vi "QD_Main.vi"(0 "State_and_Data_In":T1, 1 "Max_Queue_Size_In":i32=-1, 2 "Queue_Name_In":string, 5 "State_and_Data_N_In":T1[](array[typedef]), 7 "Time_Out_In_ms (-1)":i32, 11 "Error_In":errorcluster, 13 "Queue_Operation":T2=enum."Flush") -> (4 "State_and_Data_Out":T1, 6 "State_and_Data_N_Out":T1[](array[typedef]), 15 "Error_Out":errorcluster)   [LabVIEW 2021]
doc: "Used to transfer data from one loop to another using queue."
uses:
  Controls/State_and_Data.ctl
  Controls/Queue_Operation.ctl
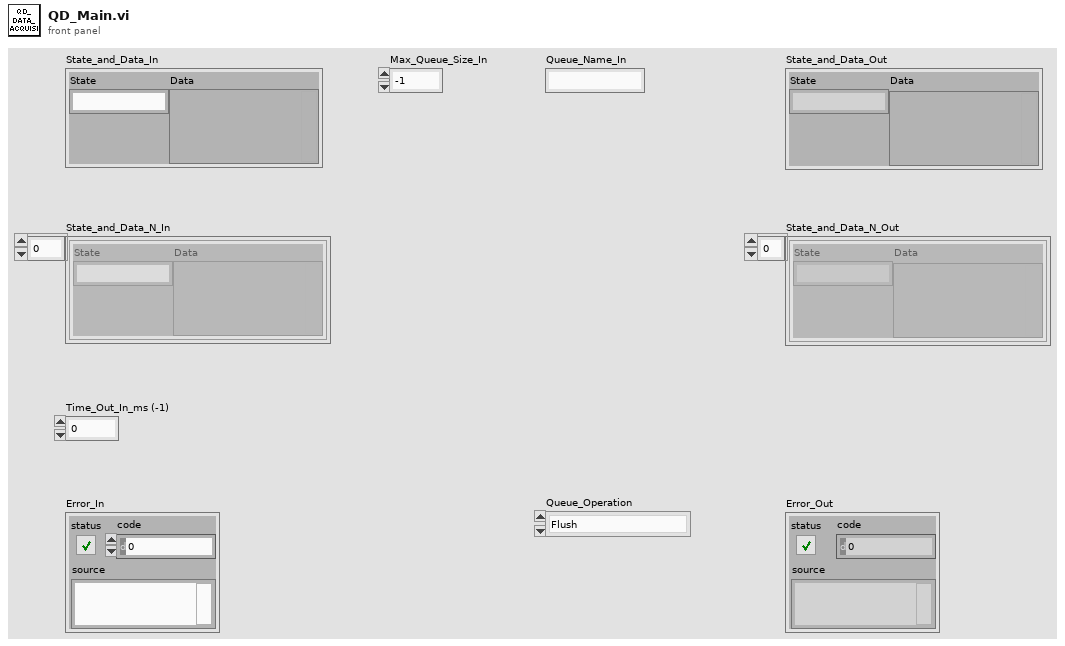
[diagram p1: front panel]
types:
  T1 = typedef "State_and_Data.ctl" = cluster{"State":string, "Data":variant}
  T2 = typedef "Queue_Operation.ctl" = enum16{"Obtain_Queue", "Enqueue", "Enqueue_First", "Enqueue_N", "Lossy_Enqueue", "Preview", "Queue_Status", "Dequeue", "Flush", "Release_Queue"}
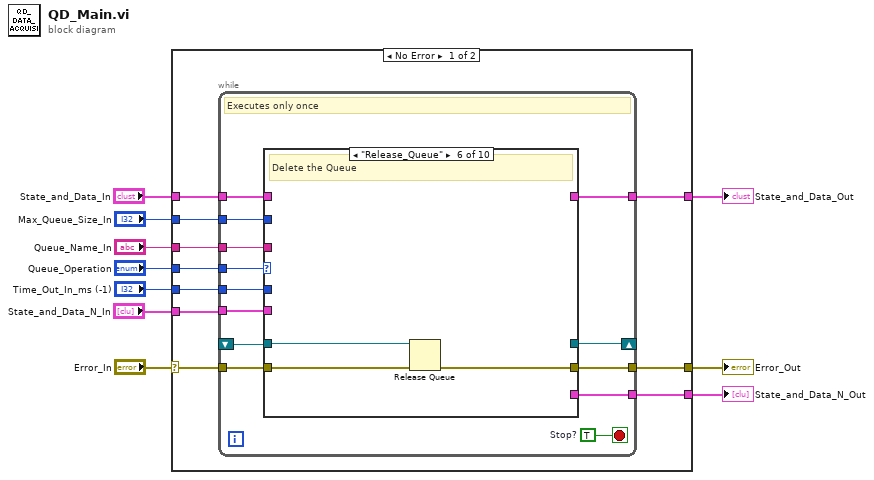
[diagram p0: block diagram]
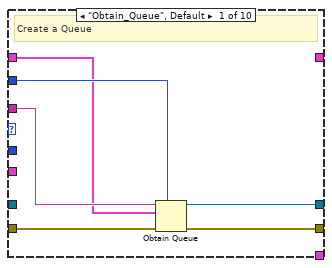
[diagram p2: hidden frame]
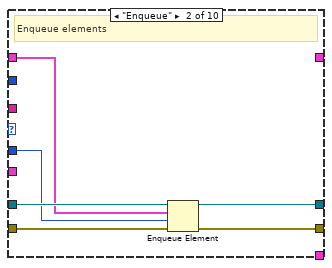
[diagram p3: hidden frame]
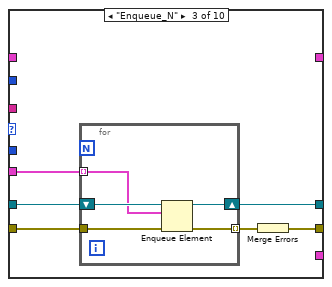
[diagram p4: hidden frame]
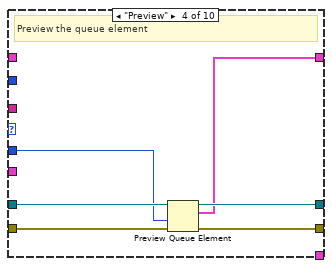
[diagram p5: hidden frame]
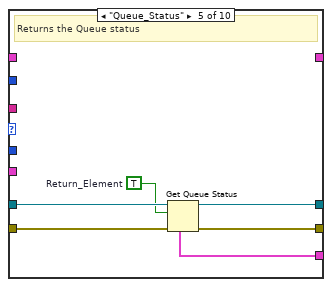
[diagram p6: hidden frame]
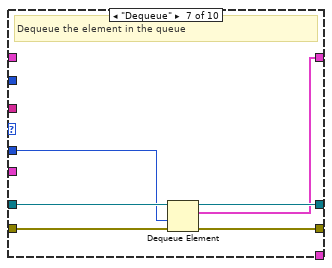
[diagram p7: hidden frame]
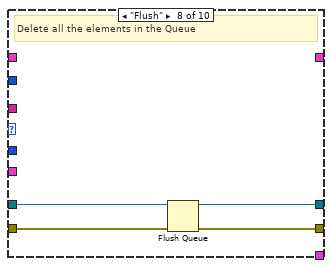
[diagram p8: hidden frame]
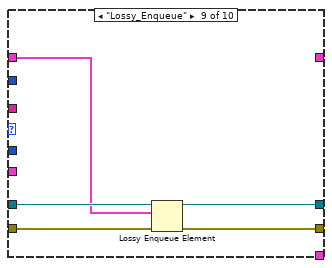
[diagram p9: hidden frame]
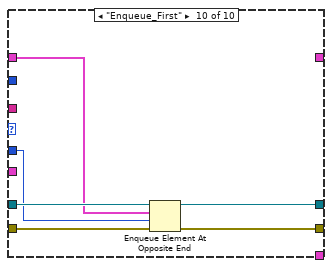
[diagram p10: hidden frame]
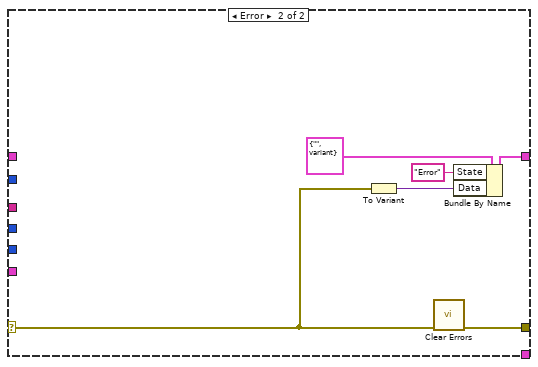
[diagram p11: hidden frame]
diagram:
  n1 = case shown="No Error" "Error_In" {
    selector: "Error_In" -> [w11 w95]
    tunnel: "Max_Queue_Size_In" -> [w20 _]
    tunnel: [w19 w98] -> w9
    tunnel: "Time_Out_In_ms (-1)" -> [w18 _]
    tunnel: "Queue_Operation" -> [w17 _]
    tunnel: "Queue_Name_In" -> [w16 _]
    tunnel: "State_and_Data_In" -> [w15 _]
    tunnel: [w14 w96] -> w4
    tunnel: [w13 _] -> w3
    tunnel: "State_and_Data_N_In" -> [w12 _]
    frame No Error {
      n2 = while {
        tunnel: w20 -> [w33]
        tunnel: w18 -> [w30]
        tunnel: w17 -> [w27]
        tunnel: [w25] -> w13
        shift-right: [w28] -> _
        shift-left: _ -> [w23]
        tunnel: w11 -> [w24]
        tunnel: [w32] -> w19
        tunnel: w12 -> [w21]
        tunnel: w16 -> [w26]
        tunnel: w15 -> [w31]
        tunnel: [w29] -> w14
        stop <- w22 stop-if-true
        w22 = TRUE  # Stop?
        # "Executes only once"
        n3 = case shown="\"Release_Queue\"" w27 {
          tunnel: w24 -> [w39 w45 w51 w61 w67 w70 w76 w80 w85 w92]
          tunnel: w26 -> [w37 _ _ _ _ _ _ _ _ _]
          tunnel: w33 -> [w36 _ _ _ _ _ _ _ _ _]
          tunnel: [w34 w41 w48 w60 w66 _ w75 w79 w84 w89] -> w28
          tunnel: [w38 w44 w46 w59 w65 w69 w73 w78 w83 w91] -> w32
          tunnel: w23 -> [_ w43 w49 w62 w68 w71 w77 w81 w86 w90]
          tunnel: w31 -> [w35 w42 _ _ _ _ _ _ w82 w88]
          tunnel: w30 -> [_ w40 _ w58 _ _ w72 _ _ w87]
          tunnel: [_ _ _ w57 _ _ w74 _ _ _] -> w29
          tunnel: [_ _ _ _ w64 _ _ _ _ _] -> w25
          tunnel: w21 -> [_ _ w47 _ _ _ _ _ _ _]
          frame "Obtain_Queue", Default {
            # "Create a Queue"
            n4 = Obtain Queue(max queue size (-1, unlimited)=w36, name (unnamed)=w37, element data type=w35, error in (no error)=w39) -> (queue out=w34:refnum<queue>, error out=w38:errorcluster)  [unwired: 1 in, 1 out]
          }
          frame "Enqueue" {
            # "Enqueue elements"
            n5 = Enqueue Element(queue=w43, element=w42, timeout in ms (-1)=w40, error in (no error)=w45) -> (queue out=w41:refnum<queue>, error out=w44:errorcluster)  [unwired: 1 out]
          }
          frame "Enqueue_N" {
            n6 = for {
              tunnel: w47 -> [w52] mode=indexing
              tunnel: w51 -> [w56]
              tunnel: [w55] -> w50 mode=indexing
              shift-right: [w53] -> w48
              shift-left: w49 -> [w54]
              n7 = Enqueue Element(queue=w54, element=w52, error in (no error)=w56) -> (queue out=w53:refnum<queue>, error out=w55:errorcluster)  [unwired: 1 in, 1 out]
            }
            n8 = Merge Errors(w50) -> (w46:errorcluster)
          }
          frame "Preview" {
            # "Preview the queue element"
            n9 = Preview Queue Element(queue=w62, timeout in ms (-1)=w58, error in (no error)=w61) -> (queue out=w60:refnum<queue>, element=w57:T1, error out=w59:errorcluster)  [unwired: 1 out]
          }
          frame "Queue_Status" {
            w63 = TRUE  # Return_Element
            # "Returns the Queue status"
            n10 = Get Queue Status(queue=w68, return elements? (F)=w63, error in (no error)=w67) -> (queue out=w66:refnum<queue>, error out=w65:errorcluster, elements=w64:T1[])  [unwired: 5 out]
          }
          frame "Release_Queue" {
            # "Delete the Queue"
            n11 = Release Queue(queue=w71, error in (no error)=w70) -> (error out=w69:errorcluster)  [unwired: 1 in, 2 out]
          }
          frame "Dequeue" {
            # "Dequeue the element in the queue"
            n12 = Dequeue Element(queue=w77, timeout in ms (-1)=w72, error in (no error)=w76) -> (queue out=w75:refnum<queue>, element=w74:T1, error out=w73:errorcluster)  [unwired: 1 out]
          }
          frame "Flush" {
            # "Delete all the elements in the Queue"
            n13 = Flush Queue(queue=w81, error in (no error)=w80) -> (queue out=w79:refnum<queue>, error out=w78:errorcluster)  [unwired: 1 out]
          }
          frame "Lossy_Enqueue" {
            n14 = Lossy Enqueue Element(queue=w86, element=w82, error in (no error)=w85) -> (queue out=w84:refnum<queue>, error out=w83:errorcluster)  [unwired: 2 out]
          }
          frame "Enqueue_First" {
            n15 = Enqueue Element At Opposite End(queue=w90, element=w88, timeout in ms (-1)=w87, error in (no error)=w92) -> (queue out=w89:refnum<queue>, error out=w91:errorcluster)  [unwired: 1 out]
          }
        }
      }
    }
    frame Error {
      n16 = To Variant(anything=w95) -> (Variant=w94:variant)
      n17 = call <vilib>:"Clear Errors.vi"("error in (no error)"=w95) -> ("error out"=w98:errorcluster)  [unwired: 5 in, 1 out]
      n18 = Bundle By Name(cluster=T1 {"State"="", "Data"=variant} ("State_and_Data_In"), "State"="Error", "Data"=w94) -> (w96:T1)
    }
  }
  "Error_Out" <- w9
  "State_and_Data_Out" <- w4
  "State_and_Data_N_Out" <- w3
